vi "RG Fetch Waveforms from scope.vi"(8 "error in (no error)":errorcluster, 9 "Maximum Time (10000ms)":u32=10000, 10 "Channels":u16[](array[ring]) items=["Channel 1", "Channel 2", "Channel 3", "Channel 4", "Math", "Reference 1", "Reference 2", "Reference 3", "Reference 4", "D0", "D1", "D2", "D3", "D4", "D5", "D6", "D7", "D8", "D9", "D10", "D11", "D12", "D13", "D14", "D15", "Amplitude", "Frequency", "Phase", "Normal", "Average", "Maximum Peak Hold", "Minimum Peak Hold"], 11 "VISA resource name":refnum<visa-resource-name>) -> (0 "error out":errorcluster, 2 "Waveform Data":waveform(dbl)[](graph), 3 "VISA resource name out":refnum<visa-resource-name>)   [LabVIEW 2017, in "Scope.lvlib" / "Tektronix DPO MSO 2000 4000 Series.lvlib"]
doc: "Initiates an acquisition on all channels that you enabled with the <B>Configure Channel</B> VI. The VI waits for the acquisition to complete and returns the waveform for the <B>Channels</B> you specified. The <B>Timeout</B> control specifies the maximum time to wait for operation complete in milliseconds. If the oscilloscope did not complete the acquisition within the time period you specify with the Timeout parameter, the VI returns a timeout error. A common cause for a timeout error is the acquisition was not triggered. For example, the trigger level is out of range of the waveform."
uses:
  Tektronix DPO MSO 2000 4000 Series.lvlib
  Data_Low Level/RG Fetch Waveform (Waveform Data Type) with delay.vi
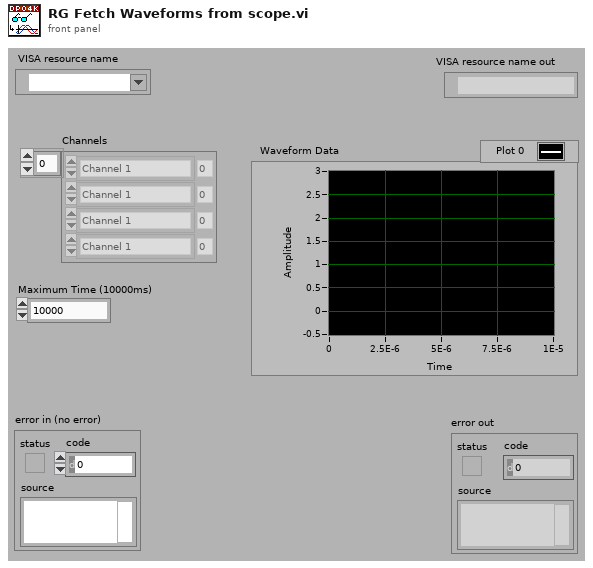
[diagram p1: front panel]
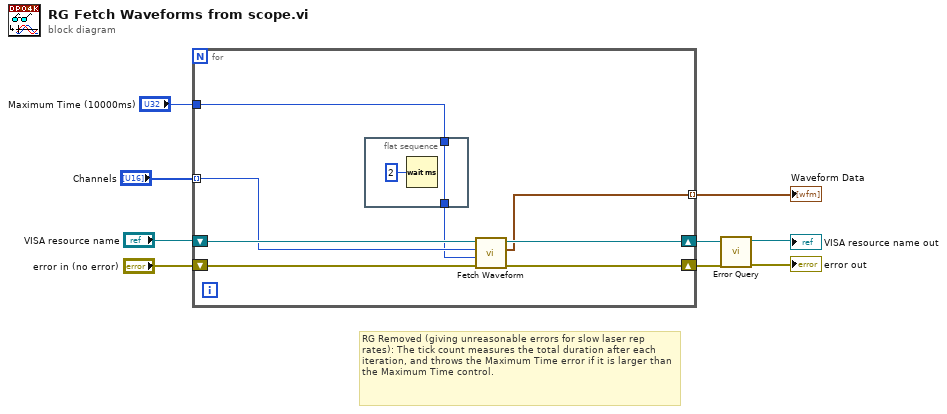
[diagram p0: block diagram]
diagram:
  # "RG Removed (giving unreasonable errors for slow laser rep rates): The tick count measures the total duration after each iteration, and throws the Maximum Time error if it is larger than the Maximum Time control."
  n1 = for {
    shift-right: [w15] -> w8
    shift-left: "VISA resource name" -> [w16]
    shift-right: [w14] -> w7
    shift-left: "error in (no error)" -> [w17]
    tunnel: "Channels" -> [w13] mode=indexing
    tunnel: [w12] -> w4 mode=indexing
    tunnel: "Maximum Time (10000ms)" -> [w11]
    n2 = flat-sequence {
      tunnel: w11 -> [w19]
      tunnel: [w19] -> w10
      frame #0 {
        n3 = Wait (ms)(milliseconds to wait=u32 2) -> ()  [unwired: 1 out]
      }
    }
    n4 = call-poly "Fetch Waveform.vi"("error in (no error)"=w17, "Maximum Time (10000ms)"=w10, "Channel (0: Channel 1)"=w13, "VISA resource name"=w16) -> ("error out"=w14:errorcluster, "Waveform Data"=w12:waveform(dbl), "VISA resource name out"=w15:refnum<visa-resource-name>)  [unwired: 5 in]
  }
  "Waveform Data" <- w4
  n5 = call "Error Query.vi"("error in (no error)"=w7, "VISA resource name"=w8) -> ("error out"=→"error out":errorcluster, "VISA resource name out"=→"VISA resource name out":refnum<visa-resource-name>)  [unwired: 6 in, 2 out]
